vi "Add Actor to DAQ Registry.vi"(8 "error in (no error)":errorcluster, 10 "Chassis Tasks out":refnum<class "Chassis Tasks.lvclass">, 11 "FP Controls in":refnum<class "FP Controls.lvclass">) -> (0 "error out":errorcluster, 3 "FP Controls out":refnum<class "FP Controls.lvclass">)   [LabVIEW 2012, in "Configuration Grandmaster.lvlib" / "FP Controls.lvclass"]
uses:
  FP Controls.lvclass
  Data Acquisition/Class Chassis Tasks/Chassis Tasks.lvclass
  FP Controls.lvclass/FP Controls.ctl
  Data Acquisition/Class Chassis Tasks/Chassis Tasks.lvclass/Chassis Tasks.ctl
  Data Acquisition/Class DAQ Task/DAQ Task.lvclass/DAQ Task.ctl
  Common/Controls/DAQ Diagnostics.ctl
  Data Acquisition/Class DAQ Task/Read Task Name.vi
  Data Acquisition/Class Chassis Tasks/Read HS DAQ Task.vi
  Data Acquisition/Class Chassis Tasks/Read LS DAQ Task.vi
  Data Acquisition/Class DAQ Task/DAQ Task.lvclass
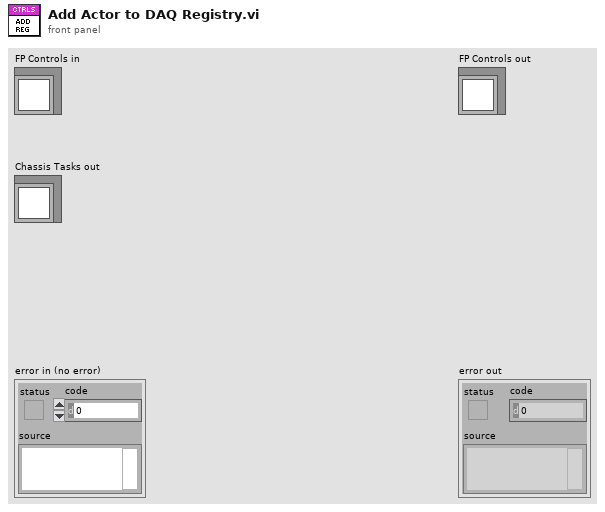
[diagram p1: front panel]
types:
  T1 = typedef "DAQ Diagnostics.ctl" = cluster{"New":bool, "LoopRate (ms)":u32, "Bff Bcklg":dbl}
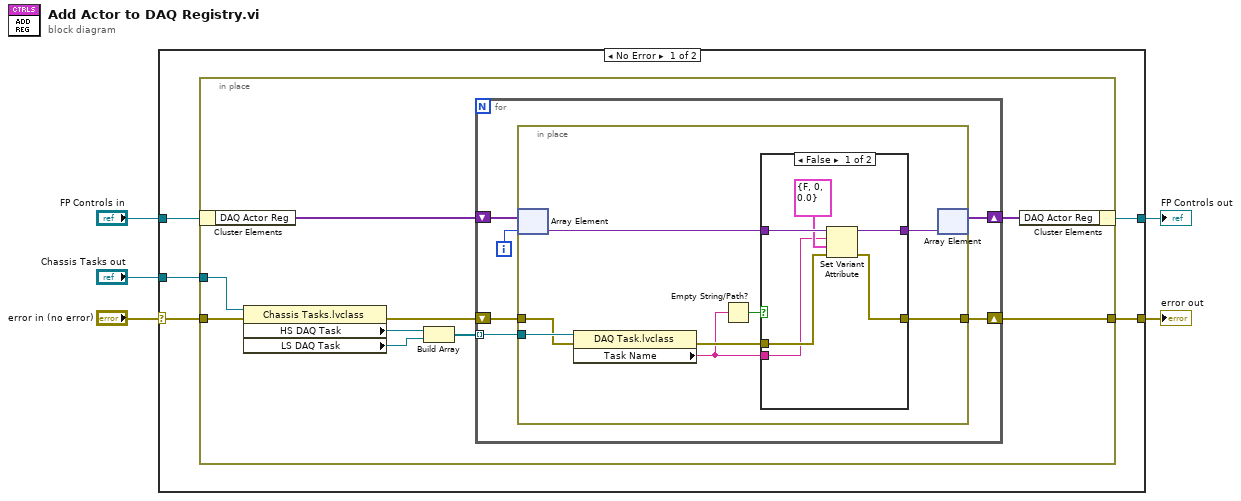
[diagram p0: block diagram]
diagram:
  n1 = case shown="No Error" "error in (no error)" {
    selector: "error in (no error)" -> [w7 w43]
    tunnel: [w6 w43] -> w4
    tunnel: [w9 w42] -> w2
    tunnel: "FP Controls in" -> [w10 w42]
    tunnel: "Chassis Tasks out" -> [w8 _]
    frame No Error {
      n2 = in-place {
        in-place-border: w8 -> [w19]
        in-place-border: w7 -> [w18]
        in-place-border: [w13] -> w6
        n3 = in-place-cluster #1(w10) -> ("DAQ Actor Reg"=w12:variant[])
        n4 = property class="Chassis Tasks.lvclass"(reference=w19, error in=w18) -> (error out=w14:errorcluster, "HS DAQ Task"=w17:refnum<class "DAQ Task.lvclass">, "LS DAQ Task"=w16:refnum<class "DAQ Task.lvclass">)  [unwired: 1 out]
        n5 = Build Array(w17, w16) -> (w15:refnum<class "DAQ Task.lvclass">[])
        n6 = for {
          tunnel: w15 -> [w25] mode=indexing
          shift-right: [w23] -> w13
          shift-left: w14 -> [w24]
          shift-right: [w20] -> w11
          shift-left: w12 -> [w22]
          i -> [w21]
          n7 = in-place {
            in-place-border: w25 -> [w33]
            in-place-border: w24 -> [w32]
            in-place-border: [w31] -> w23
            n8 = in-place-array #2(w22, w21) -> (w30:variant)
            n9 = property class="DAQ Task.lvclass"(reference=w33, error in=w32) -> (error out=w28:errorcluster, "Task Name"=w27:string)  [unwired: 1 out]
            n10 = Empty String/Path?(string/path=w27) -> (empty?=w26:bool)
            n11 = case shown="False" w26 {
              tunnel: w30 -> [w39 w41]
              tunnel: [w38 w41] -> w29
              tunnel: [w37 w40] -> w31
              tunnel: w28 -> [w35 w40]
              tunnel: w27 -> [w34 _]
              frame False {
                n12 = Set Variant Attribute(Variant=w39, name=w34, value=T1 {"New"=FALSE, "LoopRate (ms)"=0, "Bff Bcklg"=0.0} ("DAQ Diag"), error in=w35) -> (Variant out=w38:variant, error out=w37:errorcluster)  [unwired: 1 out]
              }
              frame True {
              }
            }
            n13 = in-place-array #2(w29) -> (w20:variant[])  [unwired: 1 out]
          }
        }
        n14 = in-place-cluster #1("DAQ Actor Reg"=w11) -> (w9:refnum<class "FP Controls.lvclass">)
      }
    }
    frame Error {
    }
  }
  "error out" <- w4
  "FP Controls out" <- w2
